vi "Main Loop.vi"(5 "Main Loop Command":T1, 7 "Loop cotrol command":T2=enum."Enqueue", 8 "error in":errorcluster, 11 "Data":variant) -> (0 "error out":errorcluster, 3 "Main Queue":refnum<queue>)   [LabVIEW 2018]
doc: "Create \"Main\" queue function global variables.\nIncludes the following functions:\n1. Initialize Queue\n2. Enqueue\n3. Insert Queue\n4. Fluse Queue\n5. Release Queue"
uses:
  Data Def/Loop Control Command.ctl
  Data Def/Main Loop Command.ctl
panel:
  # "Input"
  # "Output"
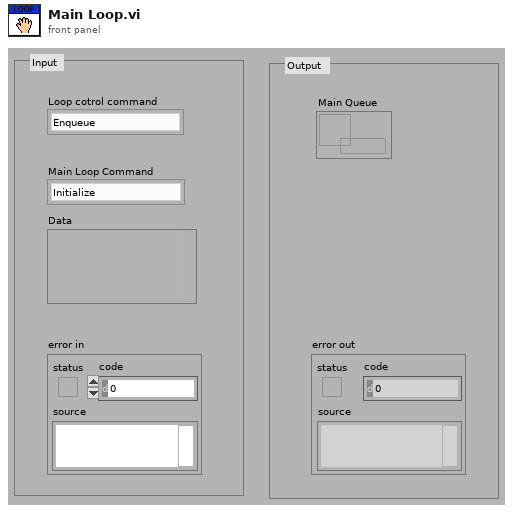
[diagram p1: front panel]
types:
  T1 = typedef "Main Loop Command.ctl" = enum16{"Initialize", "Menue", "Setting Parameter", "Get Data", "Help", "Frequency", "Channel", "Signal Type", "Previous Page", "Save", "Exit"}
  T2 = typedef "Loop Control Command.ctl" = enum16{"Initialize", "Enqueue", "Insert", "Flush", "Release"}
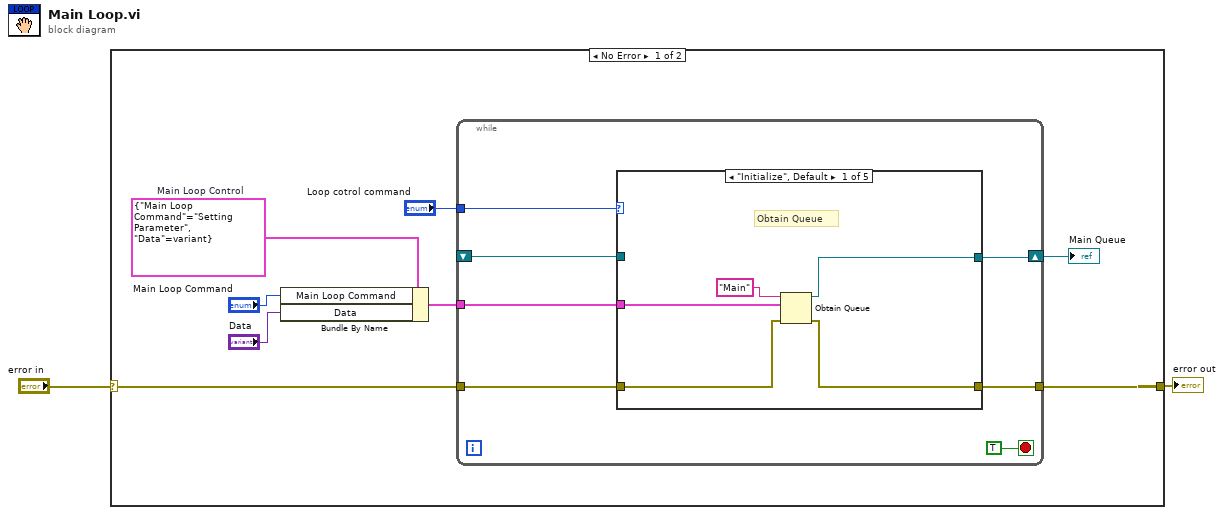
[diagram p0: block diagram]
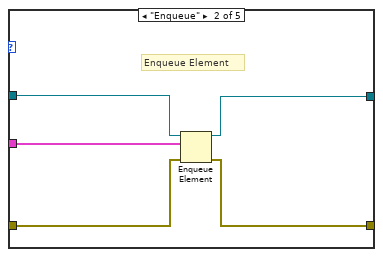
[diagram p2: hidden frame]
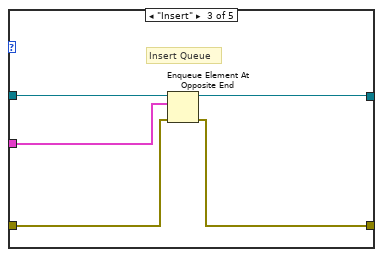
[diagram p3: hidden frame]
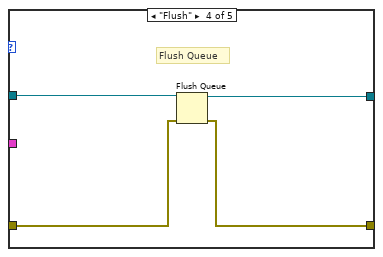
[diagram p4: hidden frame]
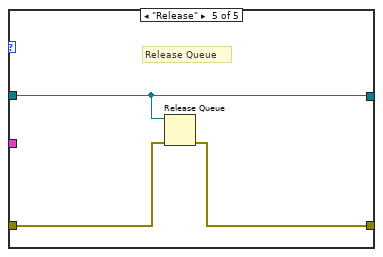
[diagram p5: hidden frame]
diagram:
  n1 = case shown="No Error" "error in" {
    selector: "error in" -> [w10 w40]
    tunnel: [w9 w40] -> w1
    frame No Error {
      w7 = cluster{"Main Loop Command":T1, "Data":variant} {"Main Loop Command"=enum."Setting Parameter", "Data"=variant}  # Main Loop Control
      n2 = Bundle By Name(cluster=w7, "Main Loop Command"="Main Loop Command", "Data"="Data") -> (w6:cluster{"Main Loop Command":T1, "Data":variant})
      n3 = while {
        tunnel: w10 -> [w17]
        tunnel: [w16] -> w9
        tunnel: "Loop cotrol command" -> [w15]
        shift-right: [w14] -> w3
        shift-left: _ -> [w12]
        tunnel: w6 -> [w13]
        stop <- TRUE stop-if-true
        n4 = case shown="\"Initialize\", Default" w15 {
          tunnel: w17 -> [w22 w24 w30 w34 w37]
          tunnel: [w21 w23 w28 w33 w39] -> w16
          tunnel: [w18 w25 w31 w35 w38] -> w14
          tunnel: w13 -> [w19 w26 w29 _ _]
          tunnel: w12 -> [_ w27 w32 w36 w38]
          frame "Initialize", Default {
            # "Obtain Queue"
            n5 = Obtain Queue(name (unnamed)="Main", element data type=w19, error in (no error)=w22) -> (queue out=w18:refnum<queue>, error out=w21:errorcluster)  [unwired: 2 in, 1 out]
          }
          frame "Enqueue" {
            # "Enqueue Element"
            n6 = Enqueue Element(queue=w27, element=w26, error in (no error)=w24) -> (queue out=w25:refnum<queue>, error out=w23:errorcluster)  [unwired: 1 in, 1 out]
          }
          frame "Insert" {
            # "Insert Queue"
            n7 = Enqueue Element At Opposite End(queue=w32, element=w29, error in (no error)=w30) -> (queue out=w31:refnum<queue>, error out=w28:errorcluster)  [unwired: 1 in, 1 out]
          }
          frame "Flush" {
            # "Flush Queue"
            n8 = Flush Queue(queue=w36, error in (no error)=w34) -> (queue out=w35:refnum<queue>, error out=w33:errorcluster)  [unwired: 1 out]
          }
          frame "Release" {
            # "Release Queue"
            n9 = Release Queue(queue=w38, error in (no error)=w37) -> (error out=w39:errorcluster)  [unwired: 1 in, 2 out]
          }
        }
      }
      "Main Queue" <- w3
    }
    frame Error {
    }
  }
  "error out" <- w1
